vi "Restore Graph Property.vi"(6 "Control Ref Queue":T1, 7 "Polor?":bool, 8 "error in (no error)":errorcluster, 11 "2D Plot.lvclass in":refnum<class "2D Plot.lvclass">) -> (0 "error out":errorcluster, 3 "2D Plot.lvclass out":refnum<class "2D Plot.lvclass">)   [LabVIEW 2017, in "2D Plot.lvclass"]
uses:
  <vilib>/Math Plots/2D Math Plots/2D Plot/2D Plot/2D Plot.lvclass
  <vilib>/Math Plots/2D Math Plots/2D Plot/Action String/2DMathPlot Ctrl Act Queue.ctl
  <vilib>/Math Plots/2D Math Plots/2D Plot/Action String/2DMathPlot Ctrl Act Cluster.ctl
  <vilib>/Math Plots/2D Math Plots/2D Plot/Action String/2DMathPlot State Class.ctl
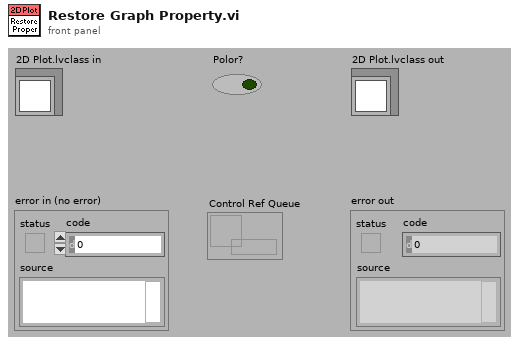
[diagram p1: front panel]
types:
  T1 = typedef "2DMathPlot Ctrl Act Queue.ctl" = refnum<queue>
  T2 = typedef "2DMathPlot State Class.ctl" = enum16{"Update All (Undo)", "Update General", "Update Appearance", "Update Format", "Update Scale", "Update Marker", "Update Cursor", "None"}
  T3 = typedef "2DMathPlot Ctrl Act Cluster.ctl" = cluster{"Plot Area Ref":refnum<vi>, "Z Axis Ref":refnum<vi>, "Legend Ref":refnum<vi>, "XControl Ref":refnum<vi>, "Facade Ref":refnum<vi>, "Display State Change Class":T2}
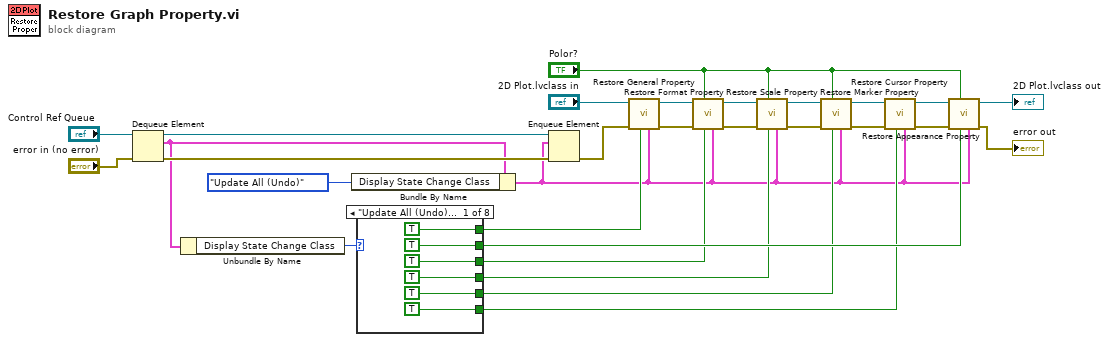
[diagram p0: block diagram]
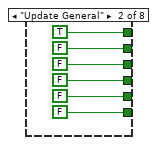
[diagram p2: hidden frame]
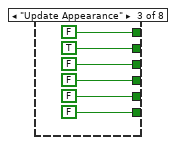
[diagram p3: hidden frame]
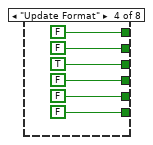
[diagram p4: hidden frame]
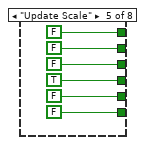
[diagram p5: hidden frame]
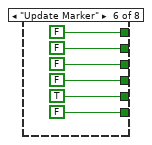
[diagram p6: hidden frame]
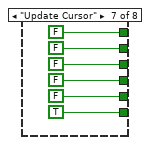
[diagram p7: hidden frame]
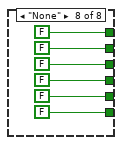
[diagram p8: hidden frame]
diagram:
  n1 = Dequeue Element(queue="Control Ref Queue", error in (no error)="error in (no error)") -> (queue out=w13:T1, element=w10:T3, error out=w12:errorcluster)  [unwired: 2 out]
  n2 = Unbundle By Name(w10) -> ("Display State Change Class"=w24:T2)
  n3 = Bundle By Name(cluster=w10, "Display State Change Class"=2DMathPlot_State_Class."Update All (Undo)") -> (w8:T3)
  n4 = case shown="\"Update All (Undo)\", Default" w24 {
    tunnel: [TRUE ("Polor?") TRUE ("Polor?") FALSE ("Polor?") FALSE ("Polor?") FALSE ("Polor?") FALSE ("Polor?") FALSE ("Polor?") FALSE ("Polor?")] -> w19
    tunnel: [TRUE ("Polor?") FALSE ("Polor?") TRUE ("Polor?") FALSE ("Polor?") FALSE ("Polor?") FALSE ("Polor?") FALSE ("Polor?") FALSE ("Polor?")] -> w18
    tunnel: [TRUE ("Polor?") FALSE ("Polor?") FALSE ("Polor?") TRUE ("Polor?") FALSE ("Polor?") FALSE ("Polor?") FALSE ("Polor?") FALSE ("Polor?")] -> w17
    tunnel: [TRUE ("Polor?") FALSE ("Polor?") FALSE ("Polor?") FALSE ("Polor?") TRUE ("Polor?") FALSE ("Polor?") FALSE ("Polor?") FALSE ("Polor?")] -> w16
    tunnel: [TRUE ("Polor?") FALSE ("Polor?") FALSE ("Polor?") FALSE ("Polor?") FALSE ("Polor?") TRUE ("Polor?") FALSE ("Polor?") FALSE ("Polor?")] -> w15
    tunnel: [TRUE ("Polor?") FALSE ("Polor?") FALSE ("Polor?") FALSE ("Polor?") FALSE ("Polor?") FALSE ("Polor?") TRUE ("Polor?") FALSE ("Polor?")] -> w14
    frame "Update All (Undo)", Default {
    }
    frame "Update General" {
    }
    frame "Update Appearance" {
    }
    frame "Update Format" {
    }
    frame "Update Scale" {
    }
    frame "Update Marker" {
    }
    frame "Update Cursor" {
    }
    frame "None" {
    }
  }
  n5 = Enqueue Element(queue=w13, element=w8, error in (no error)=w12) -> (error out=w11:errorcluster)  [unwired: 3 out]
  n6 = call <vilib>:"Restore General Property.vi"("Control Ref Cluster"=w8, "Update?"=w19, "error in (no error)"=w11, "2D Plot.lvclass in"="2D Plot.lvclass in") -> ("error out"=w2:errorcluster, "2D Plot.lvclass out"=w1:refnum<class "2D Plot.lvclass">)  [unwired: 6 out]
  n7 = call <vilib>:"Restore Format Property.vi"("Control Ref Cluster"=w8, "Update?"=w17, "Polor?"="Polor?", "error in (no error)"=w2, "2D Plot.lvclass in"=w1) -> ("error out"=w25:errorcluster, "2D Plot.lvclass out"=w26:refnum<class "2D Plot.lvclass">)  [unwired: 5 out]
  n8 = call <vilib>:"Restore Scale Property.vi"("Control Ref Cluster"=w8, "Update?"=w16, "Polor?"="Polor?", "error in (no error)"=w25, "2D Plot.lvclass in"=w26) -> ("error out"=w20:errorcluster, "2D Plot.lvclass out"=w23:refnum<class "2D Plot.lvclass">)  [unwired: 5 out]
  n9 = call <vilib>:"Restore Marker Property.vi"("Control Ref Cluster"=w8, "Update?"=w15, "Polor?"="Polor?", "error in (no error)"=w20, "2D Plot.lvclass in"=w23) -> ("error out"=w21:errorcluster, "2D Plot.lvclass out"=w22:refnum<class "2D Plot.lvclass">)  [unwired: 5 out]
  n10 = call <vilib>:"Restore Cursor Property.vi"("Control Ref Cluster"=w8, "Update?"=w14, "error in (no error)"=w21, "2D Plot.lvclass in"=w22) -> ("error out"=w4:errorcluster, "2D Plot.lvclass out"=w6:refnum<class "2D Plot.lvclass">)  [unwired: 6 out]
  n11 = call <vilib>:"Restore Appearance Property.vi"("Control Ref Cluster"=w8, "Update?"=w18, "Polor?"="Polor?", "error in (no error)"=w4, "2D Plot.lvclass in"=w6) -> ("error out"=→"error out":errorcluster, "2D Plot.lvclass out"=→"2D Plot.lvclass out":refnum<class "2D Plot.lvclass">)  [unwired: 5 out]
